vi "FTW-Benchmark-MessageTransports-PubSub.vi"() -> ()   [LabVIEW 2014]
uses:
  src/core/actor/socket/FTW-Socket-Type.ctl
  src/core/actor/socket/FTW-Socket.lvclass
  src/core/actor/subscription/FTW-Subscription.lvclass
panel:
  in  "stop":bool
  in  "Test to Perform":T1(radio)=enum."10x100x10kB"
  out "Results":T2(array[cluster]) {"?" format="%_3pB/sec (one-way receive)"; "?" format="%_3f msg/sec"; "?" format="Benchmark Time: %_3psec"}
  # "Disabled items above are due to thread limits\nin LabVIEW. This may be alleviated by directly\ncalling PostLVUserEvent from with the nanomsg\nlibrary rather than creating workers in LabVIEW\nwith blocking calls, at the expense of losing\nclient-side pushback since event queues cannot\nbe limited in LabVIEW."
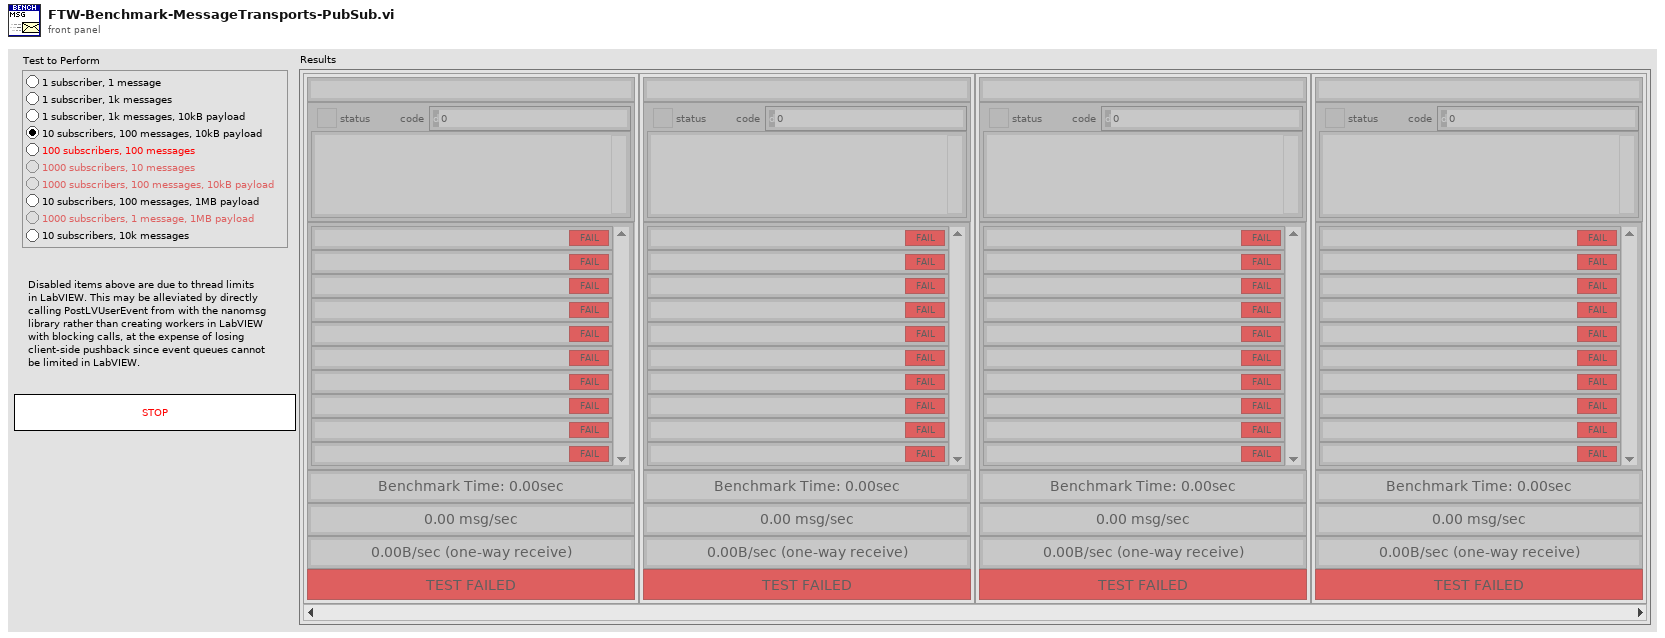
[diagram p1: front panel]
types:
  T1 = enum32{"1x1x0kB", "1x1000x0kB", "1x1000x1kB", "10x100x10kB", "100x100x0kB", "1000x10x0kB", "1000x100x10kB", "10x100x1MB", "1000x1x1MB", "10x10kx0kB"}
  T2 = cluster{"Server Address":string, "error":errorcluster, "Client Results":cluster{"Instance":string, "All replies were as expected?":bool}[], dbl, dbl, dbl, "Pass?":bool}[]
  T3 = cluster{"Inbox Address":string, "error out":errorcluster, cluster{string, bool}[], "Elapsed Time":dbl, dbl, dbl, bool}[]
  T4 = typedef "FTW-Socket.lvclass/FTW-Socket-Type.ctl" = enum32{"Server", "Client", "Publisher", "Subscriber", "Pipeline Producer", "Pipeline Consumer", "Surveyor", "Respondent", "Exclusive Pair", "Bus"}
  T5 = cluster{"Actual Endpoint Address":string, "error out":errorcluster, cluster{string, bool}[], "Elapsed Time":dbl, dbl, dbl, bool}
  T6 = cluster{"Actual Endpoint Address":string, "error out":errorcluster, cluster{string, bool}[], "Elapsed Time":dbl, dbl, dbl, bool}[]
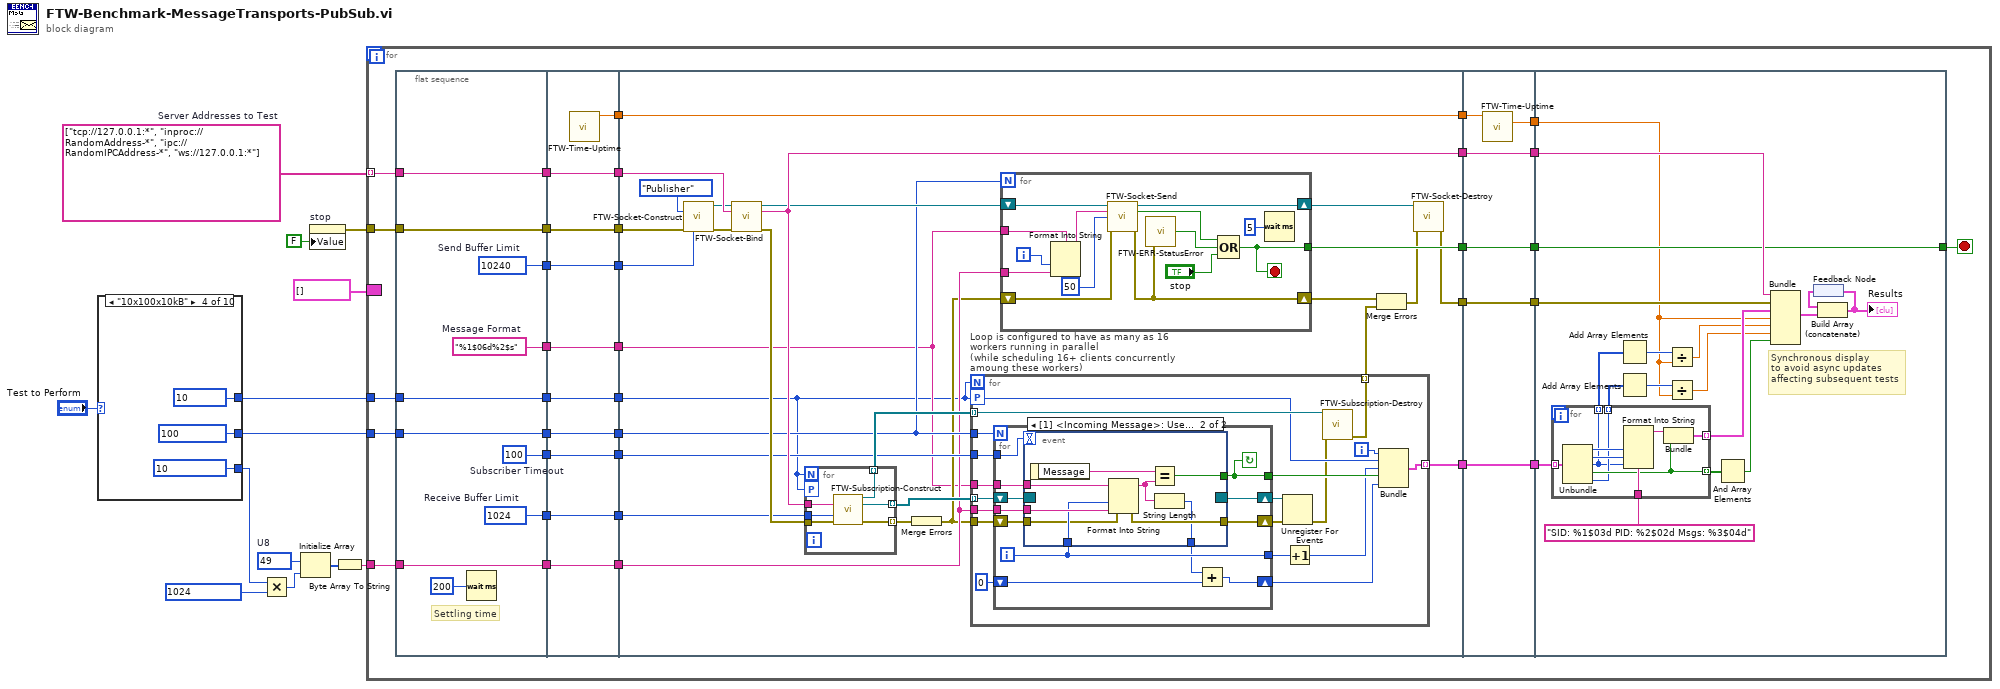
[diagram p0: block diagram]
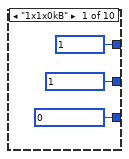
[diagram p2: hidden frame]
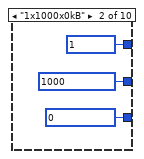
[diagram p3: hidden frame]
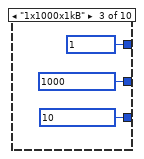
[diagram p4: hidden frame]
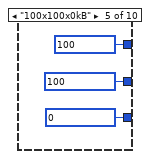
[diagram p5: hidden frame]
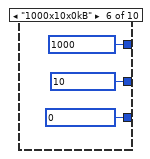
[diagram p6: hidden frame]
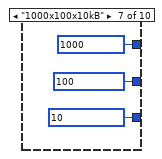
[diagram p7: hidden frame]
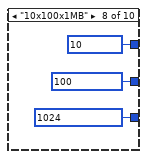
[diagram p8: hidden frame]
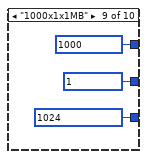
[diagram p9: hidden frame]
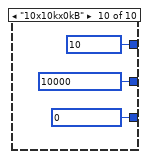
[diagram p10: hidden frame]
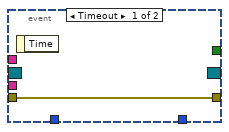
[diagram p11: hidden frame]
diagram:
  w10 = string[] ["tcp://127.0.0.1:*", "inproc://RandomAddress-*", "ipc://RandomIPCAddress-*", "ws://127.0.0.1:*"]  # Server Addresses to Test
  w13 = u8 49  # U8
  n1 = case shown="\"10x100x10kB\"" "Test to Perform" {
    tunnel: [1 1 1 10 100 1000 1000 10 1000 10] -> w8
    tunnel: [1 1000 1000 100 100 10 100 100 1 10000] -> w7
    tunnel: [0 0 10 10 0 0 10 1024 1024 0] -> w6
    frame "1x1x0kB" {
    }
    frame "1x1000x0kB" {
    }
    frame "1x1000x1kB" {
    }
    frame "10x100x10kB" {
    }
    frame "100x100x0kB" {
    }
    frame "1000x10x0kB" {
    }
    frame "1000x100x10kB" {
    }
    frame "10x100x1MB" {
    }
    frame "1000x1x1MB" {
    }
    frame "10x10kx0kB" {
    }
  }
  n2 = Multiply(x=w6, y=1024) -> (x*y=w4:i32)
  n3 = Initialize Array(w13, w4) -> (w12:u8[])
  n4 = property on="stop" class="Bool (strict)"("Value"=FALSE ("stop")) -> (error out=w1:errorcluster)  [unwired: 2 in, 1 out]
  n5 = Byte Array To String(unsigned byte array=w12) -> (string=w11:string)
  n6 = for {
    tunnel: w10 -> [w71] mode=indexing
    tunnel: w8 -> [w70]
    tunnel: w7 -> [w68]
    tunnel: w1 -> [w67]
    tunnel: w11 -> [w58]
    border: T3 [] -> [_]
    stop <- w48 stop-if-true
    n7 = flat-sequence {
      tunnel: [w88] -> w78
      tunnel: [w86] -> w72
      tunnel: w67 -> [w88]
      tunnel: w68 -> [w81]
      tunnel: w70 -> [w83]
      tunnel: w71 -> [w86]
      tunnel: [w83] -> w65
      tunnel: [w81] -> w63
      tunnel: [w84] -> w61
      tunnel: [w85] -> w59
      tunnel: w58 -> [w85]
      tunnel: [w82] -> w51
      tunnel: [w80] -> w49
      tunnel: [w79] -> w45
      tunnel: [w98] -> w77
      tunnel: [w90] -> w76
      tunnel: w78 -> [w98]
      tunnel: [w97] -> w73
      tunnel: w72 -> [w97]
      tunnel: [w96] -> w66
      tunnel: w65 -> [w96]
      tunnel: [w95] -> w64
      tunnel: w63 -> [w95]
      tunnel: [w94] -> w62
      tunnel: w61 -> [w94]
      tunnel: [w93] -> w60
      tunnel: w59 -> [w93]
      tunnel: [w92] -> w52
      tunnel: w51 -> [w92]
      tunnel: [w91] -> w50
      tunnel: w49 -> [w91]
      tunnel: w45 -> [w89]
      tunnel: [w89] -> w44
      tunnel: [w99] -> w75
      tunnel: [w125] -> w74
      tunnel: [w124] -> w69
      tunnel: w64 -> [w110]
      tunnel: w66 -> [w104]
      tunnel: w77 -> [w123]
      tunnel: w76 -> [w125]
      tunnel: w73 -> [w120]
      tunnel: w62 -> [w105]
      tunnel: w60 -> [w108]
      tunnel: [w117] -> w53
      tunnel: w52 -> [w103]
      tunnel: w50 -> [w109]
      tunnel: [w106] -> w46
      tunnel: w44 -> [w102]
      tunnel: w75 -> [w192]
      tunnel: w74 -> [w188]
      tunnel: w69 -> [w191]
      tunnel: [w192] -> w57
      tunnel: [w187] -> w56
      tunnel: [w191] -> w55
      tunnel: [w190] -> w54
      tunnel: w53 -> [w190]
      tunnel: [w189] -> w47
      tunnel: w46 -> [w189]
      tunnel: w57 -> [w209]
      tunnel: w56 -> [w195]
      tunnel: w55 -> [w208]
      tunnel: w54 -> [w210]
      tunnel: [w200] -> w48
      tunnel: w47 -> [w200]
      frame #0 {
        w80 = 100  # Subscriber Timeout
        w82 = 1024  # Receive Buffer Limit
        w79 = 10240  # Send Buffer Limit
        w84 = "%1$06d%2$s"  # Message Format
        # "Settling time"
        n8 = Wait (ms)(milliseconds to wait=u32 200) -> ()  [unwired: 1 out]
      }
      frame #1 {
        n9 = call "FTW-Time-Uptime.vi"() -> ("Current Uptime"=w90:dbl)  [unwired: 13 in, 2 out]
      }
      frame #2 {
        n10 = call "FTW-Socket-Construct.vi"("Socket Topology"=FTW-Socket-Type."Publisher", "error in"=w123, "Send Buffer Limit"=w102) -> ("FTW Socket"=w118:refnum<class "FTW-Socket.lvclass">, "error out"=w119:errorcluster)  [unwired: 11 in]
        n11 = call-dynamic "FTW-Socket-Bind.vi"("FTW Endpoint"=w118, "Remote Endpoint Address"=w120, "error in"=w119) -> ("FTW Endpoint out"=w114:refnum<class "FTW-Socket.lvclass">, "Actual Endpoint Address"=w117:string, "error out"=w116:errorcluster)  [unwired: 10 in]
        n12 = for {
          N: w104 -> [_]
          workers-P: w104 -> [_]
          tunnel: w117 -> [w131]
          tunnel: w116 -> [w130]
          tunnel: [w129] -> w112 mode=indexing
          tunnel: [w128] -> w111 mode=indexing
          tunnel: [w127] -> w115 mode=indexing
          tunnel: w103 -> [w126]
          n13 = call "FTW-Subscription-Construct.vi"("Publisher Address"=w131, "Receive Buffer Limit"=w126, "error in"=w130) -> ("FTW Subscription"=w129:refnum<class "FTW-Subscription.lvclass">, "Incoming Message"=w128:refnum<event-registration>, "error out"=w127:errorcluster)  [unwired: 10 in]
        }
        n14 = Merge Errors(w115) -> (w107:errorcluster)
        n15 = for "Loop is configured to have as many as 16 workers running in parallel\n(while scheduling 16+ clients concurrently amoung these workers)" {
          N: w104 -> [_]
          workers-P: w104 -> [w155]
          tunnel: [w164] -> w124 mode=indexing
          tunnel: [w154] -> w122 mode=indexing
          tunnel: w112 -> [w158] mode=indexing
          tunnel: w111 -> [w163] mode=indexing
          tunnel: w110 -> [w151]
          tunnel: w109 -> [w162]
          tunnel: w108 -> [w161]
          tunnel: w107 -> [w157]
          tunnel: w105 -> [w153]
          i -> [w156]
          n16 = for {
            N: w151 -> [_]
            tunnel: w162 -> [w175]
            tunnel: w161 -> [w174]
            tunnel: [w168] -> w160
            shift-right: [w171] -> w159
            shift-left: w163 -> [w176]
            shift-right: [w173] -> w149
            shift-left: w157 -> [w172]
            tunnel: w153 -> [w170]
            tunnel: [w169] -> w152
            shift-right: [w165] -> w146
            shift-left: 0 -> [w166]
            i -> [w169]
            stop <- w168 continue-if-true
            n17 = event shown="[1] <Incoming Message>: User Event" {
              selector: w176 -> [_ _]
              dyn-events: [_ _] -> w171
              timeout: w175 -> [_ _]
              tunnel: w174 -> [_ w186]
              tunnel: w169 -> [_ w185]
              tunnel: [_ w184] -> w168
              tunnel: [w177 w181] -> w173
              tunnel: w172 -> [w177 w182]
              tunnel: w170 -> [_ w183]
              tunnel: [_ w178] -> w167
              event Timeout {
                n18 = event-data() -> ()  [unwired: 1 in, 1 out]
              }
              event User Event {
                n19 = event-data() -> ("Message"=w180:string)  [unwired: 1 in]
                n20 = Format Into String(format string=w183, error in=w182, w185, w186) -> (resulting string=w179:string, error out=w181:errorcluster)  [unwired: 1 in]
                n21 = Equal?(x=w180, y=w179) -> (x = y?=w184:bool)
                n22 = String Length(string=w179) -> (length=w178:i32)
              }
            }
            n23 = Add(x=w167, y=w166) -> (x+y=w165:i32)
          }
          n24 = Unregister For Events(event registration refnum=w159, error in=w149) -> (error out=w148:errorcluster)
          n25 = Increment(x=w152) -> (x+1=w150:i32)
          n26 = call "FTW-Subscription-Destroy.vi"("FTW Subscription"=w158, "error in"=w148) -> ("error out"=w154:errorcluster)  [unwired: 13 in]
          n27 = Bundle(w156, w155, w150, w160, w146) -> (w164:cluster{i32, i32, i32, bool, i32})  [unwired: 1 in]
        }
        n28 = for {
          N: w110 -> [_]
          shift-right: [w139] -> w113
          shift-left: w114 -> [w145]
          tunnel: w108 -> [w142]
          shift-right: [w140] -> w101
          shift-left: w107 -> [w141]
          tunnel: w105 -> [w136]
          tunnel: [w135] -> w106
          i -> [w143]
          stop <- w135 stop-if-true
          n29 = Format Into String(format string=w136, w143, w142) -> (resulting string=w144:string)  [unwired: 2 in, 1 out]
          n30 = call "FTW-Socket-Send.vi"("FTW Socket"=w145, "Message"=w144, "Send Timeout"=50, "error in"=w141) -> ("FTW Socket out"=w139:refnum<class "FTW-Socket.lvclass">, "Timed out?"=w138:bool, "error out"=w140:errorcluster)  [unwired: 9 in]
          n31 = call "FTW-ERR-StatusError.vi"("error to check"=w140) -> ("Error?"=w137:bool)
          n32 = Compound Arithmetic op=OR(w138, w137, "stop") -> (w135:bool)
          n33 = Wait (ms)(milliseconds to wait=u32 5) -> ()  [unwired: 1 out]
        }
        n34 = Merge Errors(w101, w122) -> (w100:errorcluster)
        n35 = call-dynamic "FTW-Socket-Destroy.vi"("FTW Socket"=w113, "error in"=w100) -> ("error out"=w99:errorcluster)  [unwired: 13 in]
      }
      frame #3 {
        n36 = call "FTW-Time-Uptime.vi"("Previous Uptime"=w188) -> ("Elapsed Time"=w187:dbl)  [unwired: 12 in, 2 out]
      }
      frame #4 {
        # "Synchronous display\nto avoid async updates\naffecting subsequent tests"
        n37 = for {
          tunnel: w208 -> [w219] mode=indexing
          tunnel: "SID: %1$03d PID: %2$02d Msgs: %3$04d" -> [w218]
          tunnel: [w214] -> w205 mode=indexing
          tunnel: [w213] -> w207 mode=indexing
          tunnel: [w212] -> w199 mode=indexing
          tunnel: [w211] -> w198 mode=indexing
          n38 = Unbundle(w219) -> (w217:i32, w216:i32, w211:i32, w213:bool, w212:i32)
          n39 = Format Into String(format string=w218, w217, w216, w211) -> (resulting string=w215:string)  [unwired: 2 in, 1 out]
          n40 = Bundle(w215, w213) -> (w214:cluster{string, bool})  [unwired: 1 in]
        }
        n41 = Add Array Elements(numeric array=w198) -> (sum=w197:i32)
        n42 = Add Array Elements(numeric array=w199) -> (sum=w196:i32)
        n43 = Divide(x=w197, y=w195) -> (x/y=w194:dbl)
        n44 = Divide(x=w196, y=w195) -> (x/y=w193:dbl)
        n45 = And Array Elements(Boolean array=w207) -> (logical AND=w203:bool)
        n46 = Bundle("Actual Endpoint Address"=w210, "error out"=w209, w205, "Elapsed Time"=w195, w194, w193, w203) -> (w202:T5)  [unwired: 1 in]
        n47 = feedback #1() -> (w206:T3)
        n48 = Build Array (concatenate)(w206, w202) -> (w201:T6)
        "Results" <- w201
        n49 = feedback-in #1(w201) -> ()
      }
    }
  }
